vi "test22.vi"() -> ()   [LabVIEW 2012]
uses:
  freq file read-write control.ctl
panel:
  out "Array":string[](array[string])
  in  "save/read ref":refnum<vi>
  in  "save/read":T1={"write to a file list"=0, "from file "="1827_a", "clear frequency points"=FALSE, "read frequency points"=FALSE, "write frequency points"=FALSE, "to a file "="1827_a", "read from file list"=0} {"read from file list" items=["769_a", "841_a", "1399_a", "1502_a", "1527_a", "1705_a", "1916_a", "1958_a", "2061_a", "2227_a", "2365_a", "2551_a", "2713_a", "2761_a", "2964_a", "3000_a", "3030_a", "3084_a", "3235_a", "3366_a"]}
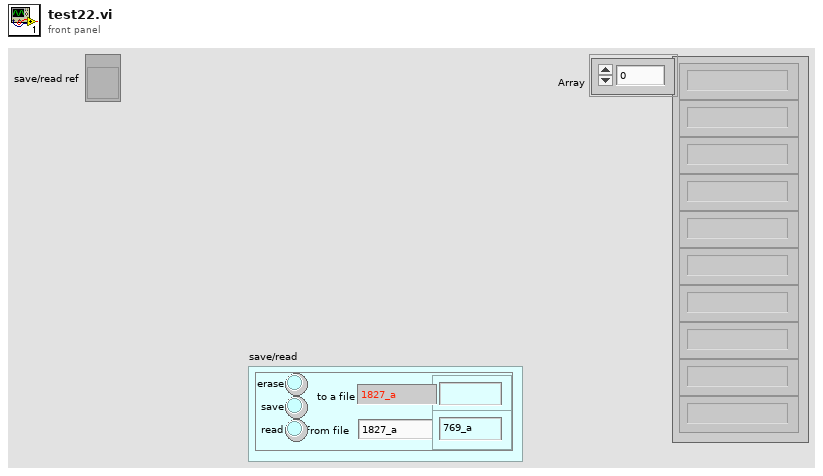
[diagram p1: front panel]
types:
  T1 = typedef "freq file read-write control.ctl" = cluster{"write to a file list":u16, "from file ":string, "clear frequency points":bool, "read frequency points":bool, "write frequency points":bool, "to a file ":string, "read from file list":u16}
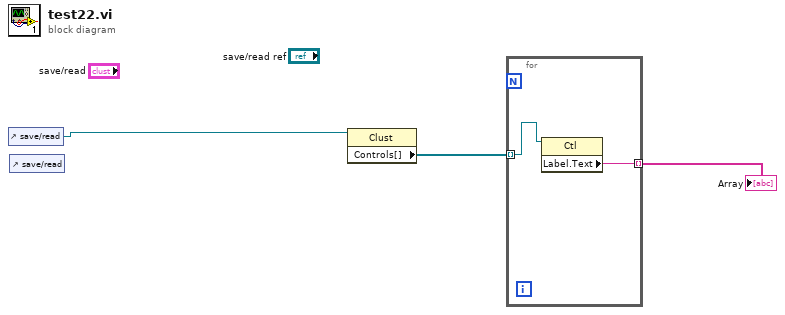
[diagram p0: block diagram]
diagram:
  n1 = control-ref of="save/read"() -> (w1:refnum<vi>)
  n2 = control-ref of="save/read"() -> ()  [unwired: 1 out]
  n3 = property class="Clust"(reference=w1) -> ("Controls[]"=w3:refnum<vi>[])  [unwired: 1 in, 2 out]
  n4 = for {
    tunnel: w3 -> [w5] mode=indexing
    tunnel: [w4] -> w2 mode=indexing
    n5 = property class="Ctl"(reference=w5) -> ("Label.Text"=w4:string)  [unwired: 1 in, 2 out]
  }
  "Array" <- w2
